vi "Read Multiple Current Measurements.vi"(8 "error in (no error)":errorcluster, 10 "Multiple Current Measurement Type (0:DC)":u16(ring) items=["DC", "Current Harmonic Amplitude", "Current Harmonic Phase", "Neutral DC Current", "Neutral Current Harmonic Amplitude", "Neutral Current Harmonic Phase"], 11 "VISA resource name":refnum<visa-resource-name>) -> (0 "error out":errorcluster, 2 "Current Measurements":sgl[](array[numeric]), 3 "VISA resource name out":refnum<visa-resource-name>)   [LabVIEW 2013, in "California Instruments iX Series.lvlib"]
doc: "Reads multiple current measurement by user selected measurement type."
uses:
  California Instruments iX Series.lvlib
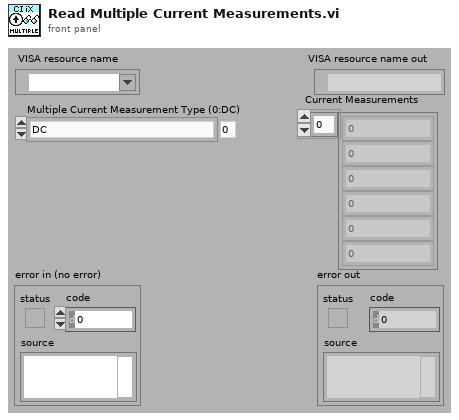
[diagram p1: front panel]
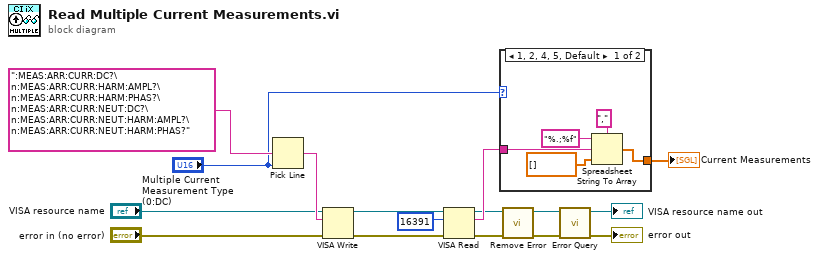
[diagram p0: block diagram]
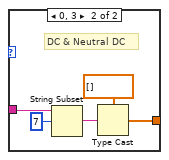
[diagram p2: hidden frame]
diagram:
  n1 = Pick Line(multi-line string=":MEAS:ARR:CURR:DC?\n:MEAS:ARR:CURR:HARM:AMPL?\n:MEAS:ARR:CURR:HARM:PHAS?\n:MEAS:ARR:CURR:NEUT:DC?\n:MEAS:ARR:CURR:NEUT:HARM:AMPL?\n:MEAS:ARR:CURR:NEUT:HARM:PHAS?", line index="Multiple Current Measurement Type (0:DC)") -> (output string=w10:string)  [unwired: 1 in]
  n2 = VISA Write(VISA resource name="VISA resource name", write buffer=w10, error in (no error)="error in (no error)") -> (VISA resource name out=w14:refnum<visa-resource-name>, error out=w13:errorcluster)  [unwired: 1 out]
  n3 = VISA Read(VISA resource name=w14, byte count=u32 16391, error in (no error)=w13) -> (VISA resource name out=w5:refnum<visa-resource-name>, read buffer=w9:string, error out=w4:errorcluster)  [unwired: 1 out]
  n4 = case shown="1, 2, 4, 5, Default" "Multiple Current Measurement Type (0:DC)" {
    tunnel: w9 -> [w21 w26]
    tunnel: [w18 w22] -> w1
    frame 1, 2, 4, 5, Default {
      n5 = Spreadsheet String To Array(delimiter (Tab)=",", format string="%.;%f", spreadsheet string=w21, array type (2D Dbl)=sgl[] []) -> (array=w18:sgl[])
    }
    frame 0, 3 {
      # "DC & Neutral DC"
      n6 = String Subset(string=w26, offset (0)=7) -> (substring=w24:string)  [unwired: 1 in]
      n7 = Type Cast(type=sgl[] [], x=w24) -> (*(type *) &x=w22:sgl[])
    }
  }
  "Current Measurements" <- w1
  n8 = call "Remove Error.vi"("error in (no error)"=w4, "VISA resource name"=w5) -> ("error out"=w6:errorcluster, "VISA resource name out"=w7:refnum<visa-resource-name>)  [unwired: 8 in]
  n9 = call "Error Query.vi"("error in (no error)"=w6, "VISA resource name"=w7) -> ("error out"=→"error out":errorcluster, "VISA resource name out"=→"VISA resource name out":refnum<visa-resource-name>)  [unwired: 6 in, 2 out]
